vi "Parse Verbose.vi"(8 "error in":errorcluster, 10 "Heartbeat in":string, 11 "Kronos in":refnum<class "Kronos.lvclass">) -> (0 "error out":errorcluster, 3 "Kronos out":refnum<class "Kronos.lvclass">)   [LabVIEW 2018, in "Kronos.lvlib" / "Kronos.lvclass"]
uses:
  Kronos.lvclass
  Custom Controls/Heartbeat Status.ctl
  Kronos.lvclass/Kronos.ctl
  Kronos.lvlib
  PPLs/Laser/Parent/Laser.lvlibp/Laser.lvclass
  C:/AME Test Engineering/LabVIEW/PPLs/Laser/Parent/Laser.lvlibp/Laser.lvclass
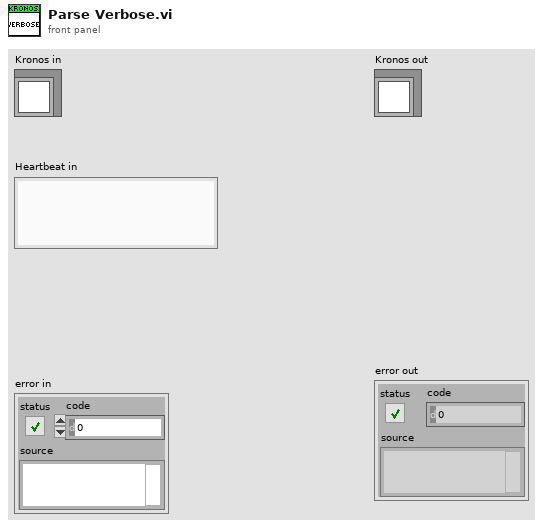
[diagram p1: front panel]
types:
  T1 = typedef "Kronos.lvlib/Heartbeat Status.ctl" = cluster{"Laser Status":bool, "On Time":dbl, "State":string, "Input Voltage":dbl, "Case Temp °C":dbl, "Board Temp °C":dbl, "Seed Temp °C":dbl, "PumpTemp °C":dbl, "Pulse Frequency (Hz)":u32, "Output Power (mW)":dbl}
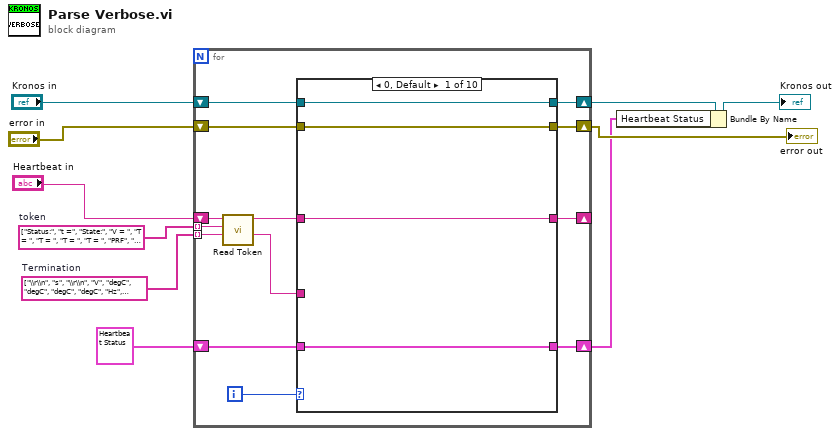
[diagram p0: block diagram]
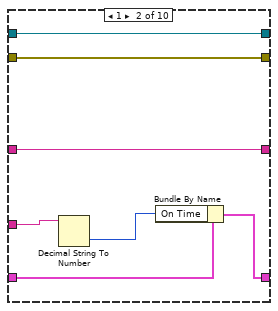
[diagram p2: hidden frame]
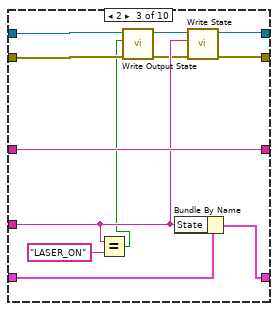
[diagram p3: hidden frame]
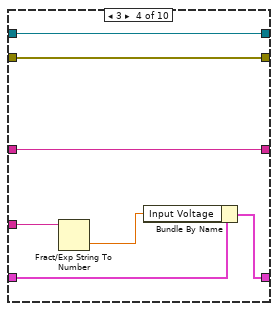
[diagram p4: hidden frame]
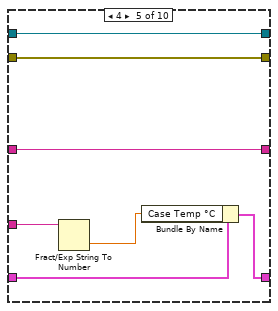
[diagram p5: hidden frame]
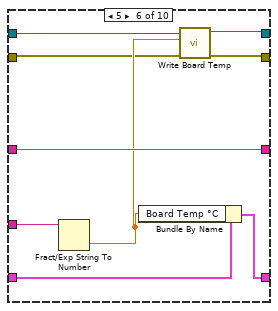
[diagram p6: hidden frame]
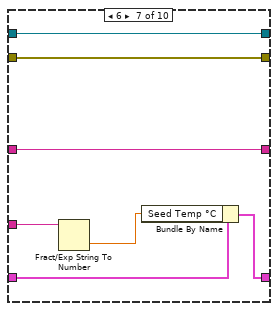
[diagram p7: hidden frame]
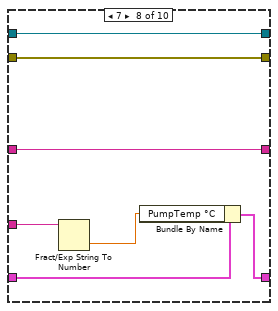
[diagram p8: hidden frame]
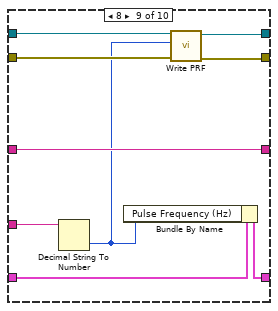
[diagram p9: hidden frame]
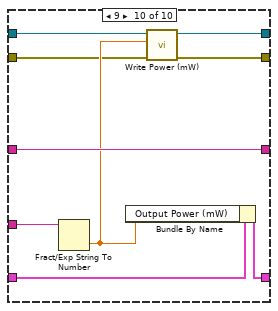
[diagram p10: hidden frame]
diagram:
  w8 = string[] ["\\r\\n", "s", "\\r\\n", "V", "degC", "degC", "degC", "degC", "Hz", "mW"]  # Termination
  w9 = string[] ["Status:", "t =", "State:", "V = ", "T = ", "T = ", "T = ", "T = ", "PRF", "P ="]  # token
  n1 = for {
    shift-right: [w15] -> _
    shift-left: "Heartbeat in" -> [w23]
    tunnel: w9 -> [w22] mode=indexing
    tunnel: w8 -> [w21] mode=indexing
    shift-right: [w18] -> w1
    shift-left: T1 {"Laser Status"=FALSE, "On Time"=0.0, "State"="", "Input Voltage"=0.0, "Case Temp °C"=0.0, "Board Temp °C"=0.0, "Seed Temp °C"=0.0, "PumpTemp °C"=0.0, "Pulse Frequency (Hz)"=0, "Output Power (mW)"=0.0} ("Heartbeat out") -> [w19]
    shift-right: [w13] -> w5
    shift-left: "Kronos in" -> [w14]
    shift-right: [w11] -> w3
    shift-left: "error in" -> [w12]
    i -> [w20]
    n2 = call "Read Token.vi"("Termination"=w21, "Token"=w22, "Status In"=w23) -> ("Parsed Value"=w17:string, "Status out"=w16:string)  [unwired: 7 in]
    n3 = case shown="0, Default" w20 {
      tunnel: w19 -> [w27 w34 w45 w53 w60 w69 w76 w83 w92 w101]
      tunnel: [w27 w33 w46 w52 w59 w68 w75 w82 w91 w100] -> w18
      tunnel: w17 -> [_ w32 w40 w51 w58 w67 w74 w81 w90 w99]
      tunnel: w16 -> [w26 w30 w44 w49 w56 w66 w72 w79 w89 w98]
      tunnel: [w26 w30 w44 w49 w56 w66 w72 w79 w89 w98] -> w15
      tunnel: w14 -> [w24 w29 w39 w47 w54 w61 w70 w77 w84 w97]
      tunnel: [w24 w29 w42 w47 w54 w64 w70 w77 w85 w96] -> w13
      tunnel: w12 -> [w25 w28 w37 w48 w55 w62 w71 w78 w88 w94]
      tunnel: [w25 w28 w43 w48 w55 w65 w71 w78 w87 w93] -> w11
      frame 0, Default {
      }
      frame 1 {
        n4 = Decimal String To Number(string=w32) -> (number=w31:i32)  [unwired: 2 in, 1 out]
        n5 = Bundle By Name(cluster=w34, "On Time"=w31) -> (w33:T1)
      }
      frame 2 {
        n6 = Equal?(x=w40, y="LASER_ON") -> (x = y?=w35:bool)
        n7 = call "Write Output State.vi"("error in (no error)"=w37, "Output State"=w35, "Laser in"=w39) -> ("error out"=w36:errorcluster, "Laser out"=w38:refnum<class "Kronos.lvclass">)  [unwired: 7 in]
        n8 = Bundle By Name(cluster=w45, "State"=w40) -> (w46:T1)
        n9 = call "Write State.vi"("error in (no error)"=w36, "State"=w40, "Laser in"=w38) -> ("error out"=w43:errorcluster, "Laser out"=w42:refnum<class "Kronos.lvclass">)  [unwired: 7 in]
      }
      frame 3 {
        n10 = Fract/Exp String To Number(string=w51) -> (number=w50:dbl)  [unwired: 3 in, 1 out]
        n11 = Bundle By Name(cluster=w53, "Input Voltage"=w50) -> (w52:T1)
      }
      frame 4 {
        n12 = Fract/Exp String To Number(string=w58) -> (number=w57:dbl)  [unwired: 3 in, 1 out]
        n13 = Bundle By Name(cluster=w60, "Case Temp °C"=w57) -> (w59:T1)
      }
      frame 5 {
        n14 = Fract/Exp String To Number(string=w67) -> (number=w63:dbl)  [unwired: 3 in, 1 out]
        n15 = Bundle By Name(cluster=w69, "Board Temp °C"=w63) -> (w68:T1)
        n16 = call "Write Board Temp.vi"("error in (no error)"=w62, "Board Temp"=w63, "Laser in"=w61) -> ("error out"=w65:errorcluster, "Laser out"=w64:refnum<class "Kronos.lvclass">)  [unwired: 7 in]
      }
      frame 6 {
        n17 = Fract/Exp String To Number(string=w74) -> (number=w73:dbl)  [unwired: 3 in, 1 out]
        n18 = Bundle By Name(cluster=w76, "Seed Temp °C"=w73) -> (w75:T1)
      }
      frame 7 {
        n19 = Fract/Exp String To Number(string=w81) -> (number=w80:dbl)  [unwired: 3 in, 1 out]
        n20 = Bundle By Name(cluster=w83, "PumpTemp °C"=w80) -> (w82:T1)
      }
      frame 8 {
        n21 = Decimal String To Number(string=w90) -> (number=w86:i32)  [unwired: 2 in, 1 out]
        n22 = Bundle By Name(cluster=w92, "Pulse Frequency (Hz)"=w86) -> (w91:T1)
        n23 = call "Write PRF.vi"("error in (no error)"=w88, "PRF"=w86, "Laser in"=w84) -> ("error out"=w87:errorcluster, "Laser out"=w85:refnum<class "Kronos.lvclass">)  [unwired: 7 in]
      }
      frame 9 {
        n24 = Fract/Exp String To Number(string=w99) -> (number=w95:dbl)  [unwired: 3 in, 1 out]
        n25 = Bundle By Name(cluster=w101, "Output Power (mW)"=w95) -> (w100:T1)
        n26 = call "Write Power (mW).vi"("error in (no error)"=w94, "Power (mW)"=w95, "Laser in"=w97) -> ("error out"=w93:errorcluster, "Laser out"=w96:refnum<class "Kronos.lvclass">)  [unwired: 7 in]
      }
    }
  }
  "error out" <- w3
  n27 = Bundle By Name(cluster=w5, "Heartbeat Status"=w1) -> (→"Kronos out":refnum<class "Kronos.lvclass">)
